vi "Post-Build Action.vi"(5 "Files Generated by Build":path[](array[path]), 6 "Top Level/Always Included VIs":path[](array[path]), 7 "Destination Path":path, 8 "error in (no error)":errorcluster, 9 "Target Name":string, 10 "Build Specification Name":string, 11 "Project Path":path) -> (0 "error out":errorcluster)   [LabVIEW 2026, in "Build VIs.lvlib"]
uses:
  Build VIs.lvlib
  <userlib>/_OpenG.lib/file/file.llb/openg_file.lvlib
  C:/Users/ppathak/Downloads/NationalInstruments.VeriStand.dll
  Users/ppathak/Downloads/NationalInstruments.VeriStand.dll
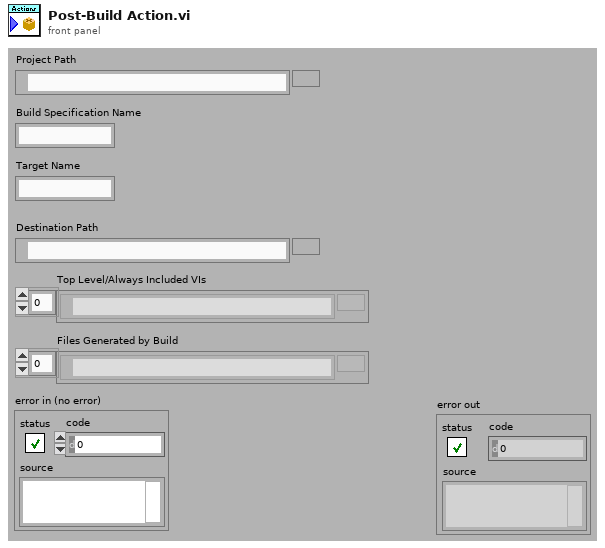
[diagram p1: front panel]
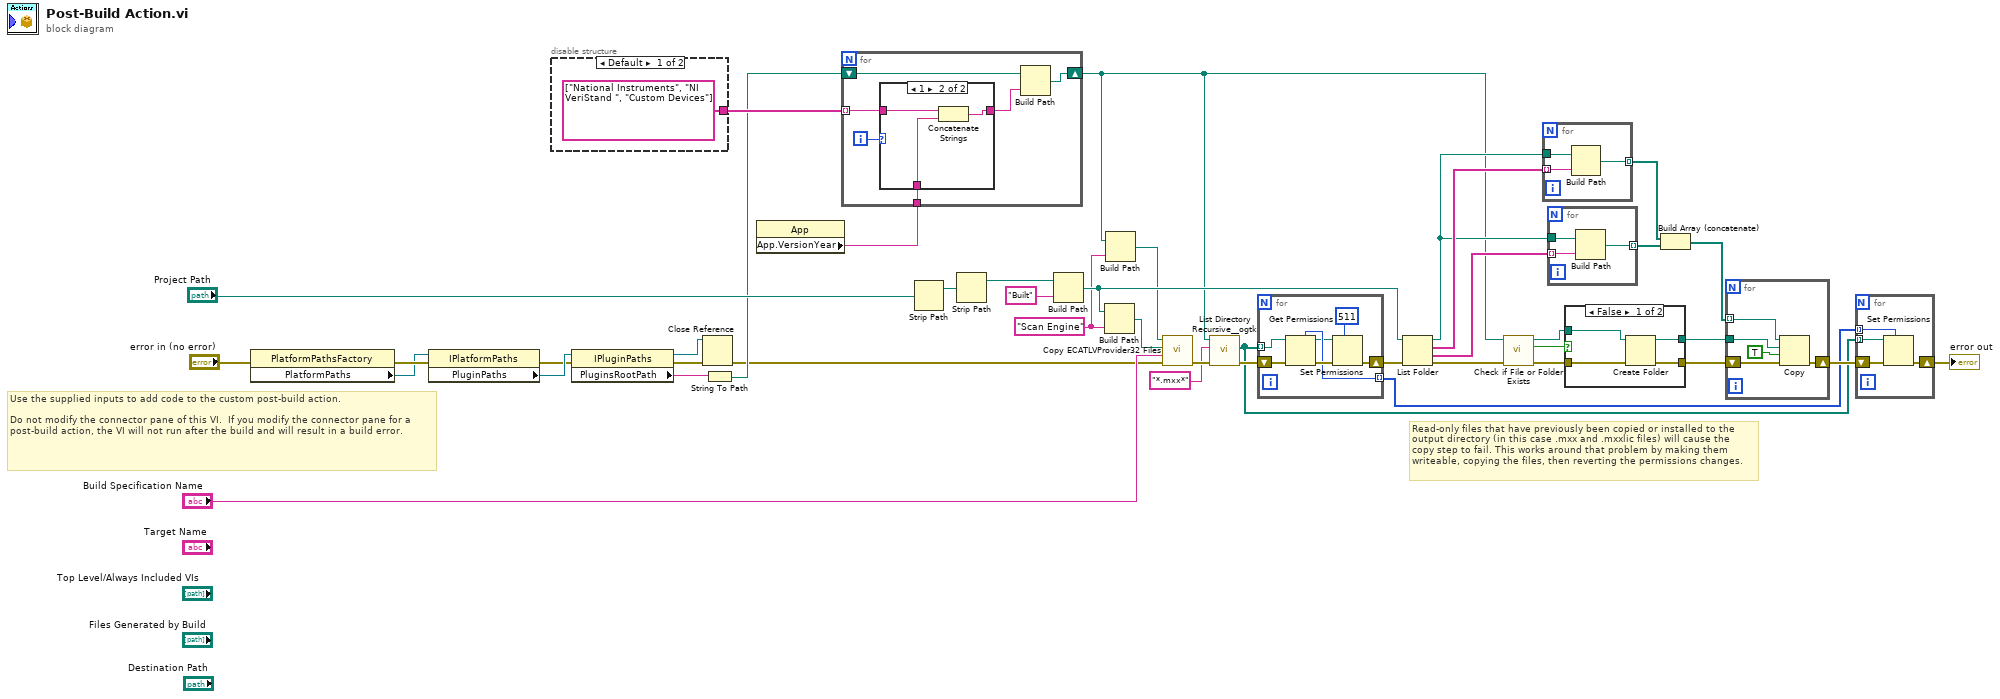
[diagram p0: block diagram]
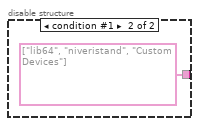
[diagram p2: hidden frame]
diagram:
  w23 = "Scan Engine" ("name or relative path")
  # "Read-only files that have previously been copied or installed to the\noutput directory (in this case .mxx and .mxxlic files) will cause the\ncopy step to fail. This works around that problem by making them\nwriteable, copying the files, then reverting the permissions changes."
  # "Use the supplied inputs to add code to the custom post-build action.\n\nDo not modify the connector pane of this VI.  If you modify the connector pane for a post-build action, the VI will not run after the build and will result in a build error."
  n1 = property class="PlatformPathsFactory"(error in="error in (no error)") -> (error out=w8:errorcluster, "PlatformPaths"=w6:refnum<k24>)  [unwired: 1 in, 1 out]
  n2 = property class="IPlatformPaths"(reference=w6, error in=w8) -> (error out=w7:errorcluster, "PluginPaths"=w9:refnum<k24>)  [unwired: 1 out]
  n3 = disable-structure shown="Default" {
    disable-tunnel: [string[] ["National Instruments", "NI VeriStand ", "Custom Devices"] string[] ["lib64", "niveristand", "Custom Devices"]] -> w26
    frame condition #0 (active) {
    }
    frame condition #1 {
    }
  }
  n4 = property class="IPluginPaths"(reference=w9, error in=w7) -> (reference out=w3:refnum<k24>, error out=w1:errorcluster, "PluginsRootPath"=w10:string)
  n5 = Close Reference(reference=w3, error in (no error)=w1) -> (error out=w2:errorcluster)
  n6 = String To Path(string=w10) -> (path=w4:path)
  n7 = property class="App"() -> ("App.VersionYear"=w25:string)  [unwired: 2 in, 2 out]
  n8 = for {
    shift-right: [w49] -> w19
    shift-left: w4 -> [w50]
    tunnel: w26 -> [w46] mode=indexing
    tunnel: w25 -> [w45]
    i -> [w48]
    n9 = case shown="1" w48 {
      tunnel: [w51 w53] -> w47
      tunnel: w46 -> [w51 w54]
      tunnel: w45 -> [_ w52]
      frame Default {
      }
      frame 1 {
        n10 = Concatenate Strings(w54, w52) -> (w53:string)
      }
    }
    n11 = Build Path(base path=w50, name or relative path=w47) -> (appended path=w49:path)
  }
  n12 = Strip Path(path="Project Path") -> (stripped path=w28:path)  [unwired: 1 out]
  n13 = Strip Path(path=w28) -> (stripped path=w38:path)  [unwired: 1 out]
  n14 = Build Path(base path=w38, name or relative path="Built") -> (appended path=w24:path)
  n15 = Build Path(base path=w24, name or relative path=w23) -> (appended path=w21:path)
  n16 = Build Path(base path=w19, name or relative path=w23) -> (appended path=w22:path)
  n17 = call "Copy ECATLVProvider32 Files.vi"("error in"=w2, "Build Specification Name"="Build Specification Name", "Source Path"=w21, "Destination Path"=w22) -> ("error out"=w20:errorcluster)  [unwired: 7 in]
  n18 = call <userlib>:"List Directory Recursive__ogtk.vi"("error in (no error)"=w20, "pattern"="*.mxx*", "Path"=w19) -> ("error out"=w17:errorcluster, "file paths"=w13:path[])  [unwired: 5 in, 2 out]
  n19 = for {
    shift-right: [w60] -> w16
    shift-left: w17 -> [w59]
    tunnel: w13 -> [w57] mode=indexing
    tunnel: [w56] -> w12 mode=indexing
    n20 = Get Permissions(8:w59, 11:w57) -> (0:w58:errorcluster, 3:w55:path, 5:w56:i16)  [unwired: 2 out]
    n21 = Set Permissions(7:i16 511 ("permissions"), 8:w58, 11:w55) -> (0:w60:errorcluster)  [unwired: 2 in, 1 out]
  }
  n22 = List Folder(path=w24, error in=w16) -> (path out=w30:path, filenames=w42:string[], folder names=w31:string[], error out=w27:errorcluster)  [unwired: 2 in]
  n23 = call <vilib>:"Check if File or Folder Exists.vi"("error in (no error)"=w27, "path"=w19) -> ("error out"=w34:errorcluster, "file or folder exists?"=w36:bool, "dup path"=w35:path)  [unwired: 7 in]
  n24 = for {
    tunnel: w42 -> [w63] mode=indexing
    tunnel: w30 -> [w64]
    tunnel: [w62] -> w41 mode=indexing
    n25 = Build Path(base path=w64, name or relative path=w63) -> (appended path=w62:path)
  }
  n26 = for {
    tunnel: w31 -> [w66] mode=indexing
    tunnel: w30 -> [w67]
    tunnel: [w65] -> w29 mode=indexing
    n27 = Build Path(base path=w67, name or relative path=w66) -> (appended path=w65:path)
  }
  n28 = case shown="False" w36 {
    tunnel: w35 -> [w71 w73]
    tunnel: w34 -> [w70 w72]
    tunnel: [w69 w73] -> w33
    tunnel: [w68 w72] -> w32
    frame False {
      n29 = Create Folder(path (use dialog)=w71, error in=w70) -> (created path=w69:path, error out=w68:errorcluster)  [unwired: 1 in, 1 out]
    }
    frame True {
    }
  }
  n30 = Build Array (concatenate)(w41, w29) -> (w40:path[])
  n31 = for {
    tunnel: w40 -> [w75] mode=indexing
    shift-right: [w76] -> w15
    shift-left: w32 -> [w77]
    tunnel: w33 -> [w74]
    n32 = Copy(8:w77, 9:TRUE ("overwrite (F)"), 10:w74, 11:w75) -> (0:w76:errorcluster)  [unwired: 1 in, 2 out]
  }
  n33 = for {
    shift-right: [w82] -> w14
    shift-left: w15 -> [w81]
    tunnel: w13 -> [w80] mode=indexing
    tunnel: w12 -> [w79] mode=indexing
    n34 = Set Permissions(7:w79, 8:w81, 11:w80) -> (0:w82:errorcluster)  [unwired: 2 in, 1 out]
  }
  "error out" <- w14
